vi "StoreUndoEntry.vi"(5 "Text.Selection":T1, 6 "Max Depth (100)":i32=100, 7 "Changed Editor":refnum<vi>, 8 "error in (no error)":errorcluster, 9 "editor refs":refnum<vi>[](array[refnum]), 10 "Tree":refnum<vi>, 11 "UndoBuffer":refnum<vi>[](array[refnum])) -> (0 "error out":errorcluster)   [LabVIEW 2020, in "ScriptManager.lvlib"]
uses:
  ScriptManager.lvlib
  <vilib>/Utility/miscctls.llb/LVSelectionTypeDef.ctl
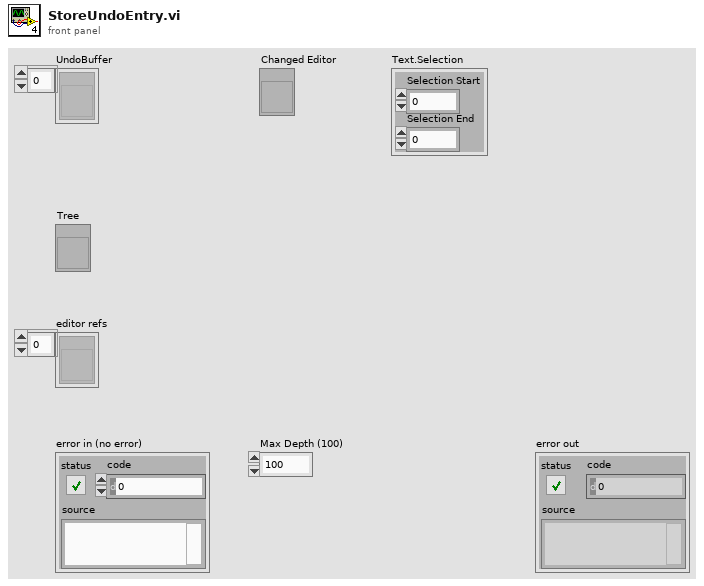
[diagram p1: front panel]
types:
  T1 = typedef "LVSelectionTypeDef.ctl" = cluster{"Selection Start":u32, "Selection End":u32}
  T2 = cluster{"UndoBuffer[0]":refnum<vi>, "UndoBuffer[1]":refnum<vi>, "UndoBuffer[2]":refnum<vi>}
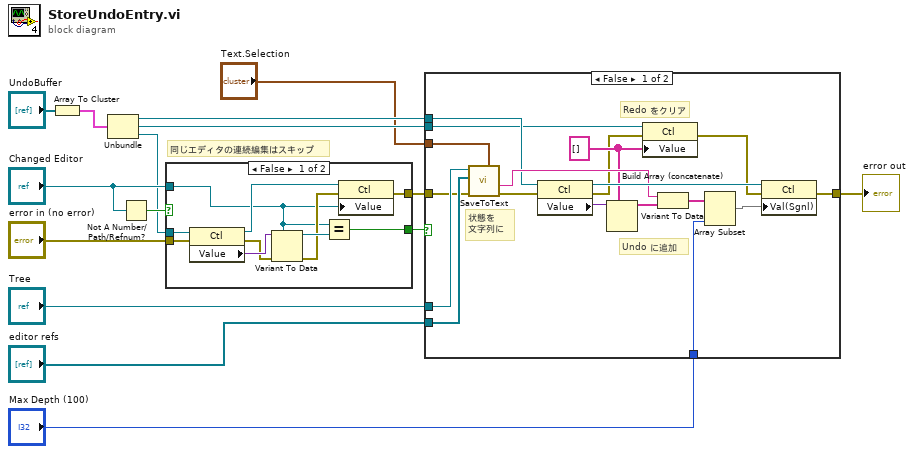
[diagram p0: block diagram]
diagram:
  # "同じエディタの連続編集はスキップ"
  n1 = Array To Cluster(array="UndoBuffer") -> (cluster=w11:T2)
  n2 = Unbundle(w11) -> ("UndoBuffer[0]"=w10:refnum<vi>, "UndoBuffer[1]"=w9:refnum<vi>, "UndoBuffer[2]"=w5:refnum<vi>)
  n3 = Not A Number/Path/Refnum?(number/path/refnum="Changed Editor") -> (NaN/Path/Refnum?=w7:bool)
  n4 = case shown="False" w7 {
    tunnel: "Changed Editor" -> [w16 _]
    tunnel: w5 -> [w25 _]
    tunnel: "error in (no error)" -> [w21 w26]
    tunnel: [w20 _] -> w3
    tunnel: [w17 w26] -> w2
    frame False {
      n5 = property class="Ctl"(reference=w25, error in=w21) -> (reference out=w19:refnum<vi>, error out=w22:errorcluster, "Value"=w24:variant)
      n6 = Variant To Data(error in=w22, type=w16, Variant=w24) -> (data=w23:refnum<vi>, error out=w18:errorcluster)
      n7 = Equal?(x=w16, y=w23) -> (x = y?=w20:bool)
      n8 = property class="Ctl"(reference=w19, error in=w18, "Value"=w16) -> (error out=w17:errorcluster)  [unwired: 1 out]
    }
    frame True {
    }
  }
  n9 = case shown="False" w3 {
    tunnel: "Tree" -> [w44 _]
    tunnel: "editor refs" -> [w43 _]
    tunnel: [w39 w45] -> w13
    tunnel: "Max Depth (100)" -> [w36 _]
    tunnel: w10 -> [w34 _]
    tunnel: w9 -> [w33 _]
    tunnel: w2 -> [w30 w45]
    tunnel: "Text.Selection" -> [w27 _]
    frame False {
      w31 = string[] [] ("Value")
      # "状態を\n文字列に"
      # "Undo に追加"
      # "Redo をクリア"
      n10 = call "SaveToText.vi"("Text.Selection"=w27, "error in (no error)"=w30, "editor refs"=w43, "Tree ref"=w44) -> ("error out"=w41:errorcluster, "String"=w35:string)  [unwired: 6 in]
      n11 = property class="Ctl"(reference=w34, error in=w41) -> (reference out=w40:refnum<vi>, error out=w29:errorcluster, "Value"=w42:variant)
      n12 = Variant To Data(type=w31, Variant=w42) -> (data=w32:string[])  [unwired: 1 in, 1 out]
      n13 = property class="Ctl"(reference=w33, error in=w29, "Value"=w31) -> (error out=w28:errorcluster)  [unwired: 1 out]
      n14 = Build Array (concatenate)(w35, w32) -> (w37:string[])
      n15 = Array Subset(array=w37, length=w36) -> (w38:string[])  [unwired: 1 in]
      n16 = property class="Ctl"(reference=w40, error in=w28, "Val(Sgnl)"=w38) -> (error out=w39:errorcluster)  [unwired: 1 out]
    }
    frame True {
    }
  }
  "error out" <- w13
